vi "Read Path Switch.lvclass.vi"(11 "PathControl in":refnum<class "PathControl.lvclass">) -> (2 "Path Switch.lvclass":refnum<class "Path Switch.lvclass">, 3 "PathControl out":refnum<class "PathControl.lvclass">)   [LabVIEW 2020, in "PathControl.lvclass"]
uses:
  PathControl.lvclass
  Instruments/Path Switch/Path Switch.lvclass
  PathControl.lvclass/PathControl.ctl
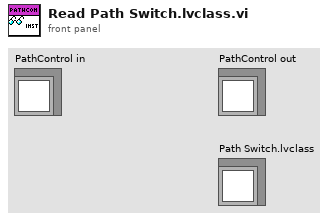
[diagram p1: front panel]
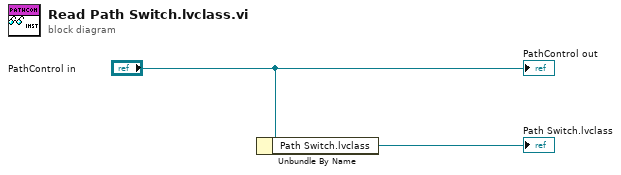
[diagram p0: block diagram]
diagram:
  n1 = Unbundle By Name("PathControl in") -> ("Path Switch.lvclass"=→"Path Switch.lvclass":refnum<class "Path Switch.lvclass">)
  "PathControl out" <- "PathControl in"
